vi "Set Hardware FP Connections.vi"(7 "command (Connect)":T8, 8 "error in (no error)":errorcluster, 11 "Engine Run Time Data in":T1) -> (0 "error out":errorcluster, 3 "Engine Run Time Data out":T1)   [LabVIEW 2023, in "NI 272x Resistive Simulation Custom Device Engine.lvlib"]
uses:
  NI 272x Resistive Simulation Custom Device Engine.lvlib
  <instrlib>/ni272xReferenceVIs/ni272xReferenceVIs.llb/ni272x Connector Identifier.ctl
  <instrlib>/ni272xReferenceVIs/ni272xReferenceVIs.llb/ni272x Disconnect from Connector 1Chan.vi
  <instrlib>/ni272xReferenceVIs/ni272xReferenceVIs.llb/ni272x Connect to Connector 1Chan.vi
  <instrlib>/ni272xReferenceVIs/ni272xReferenceVIs.llb/ni272x Reference.ctl
  Controls/Connection control.ctl
  Controls/Channel Mode.ctl
  NI 272x Resistive Simulation Custom Device Shared.lvlib
  <instrlib>/ni272xReferenceVIs/ni272xReferenceVIs.llb/ni272x Callendar-Van Dusen RTD Parameters.ctl
  Controls/Compiled HW Channel.ctl
  Controls/Compiled Connect Channel.ctl
  Controls/Compiled Engine Data.ctl
  Controls/Engine Run Time Data.ctl
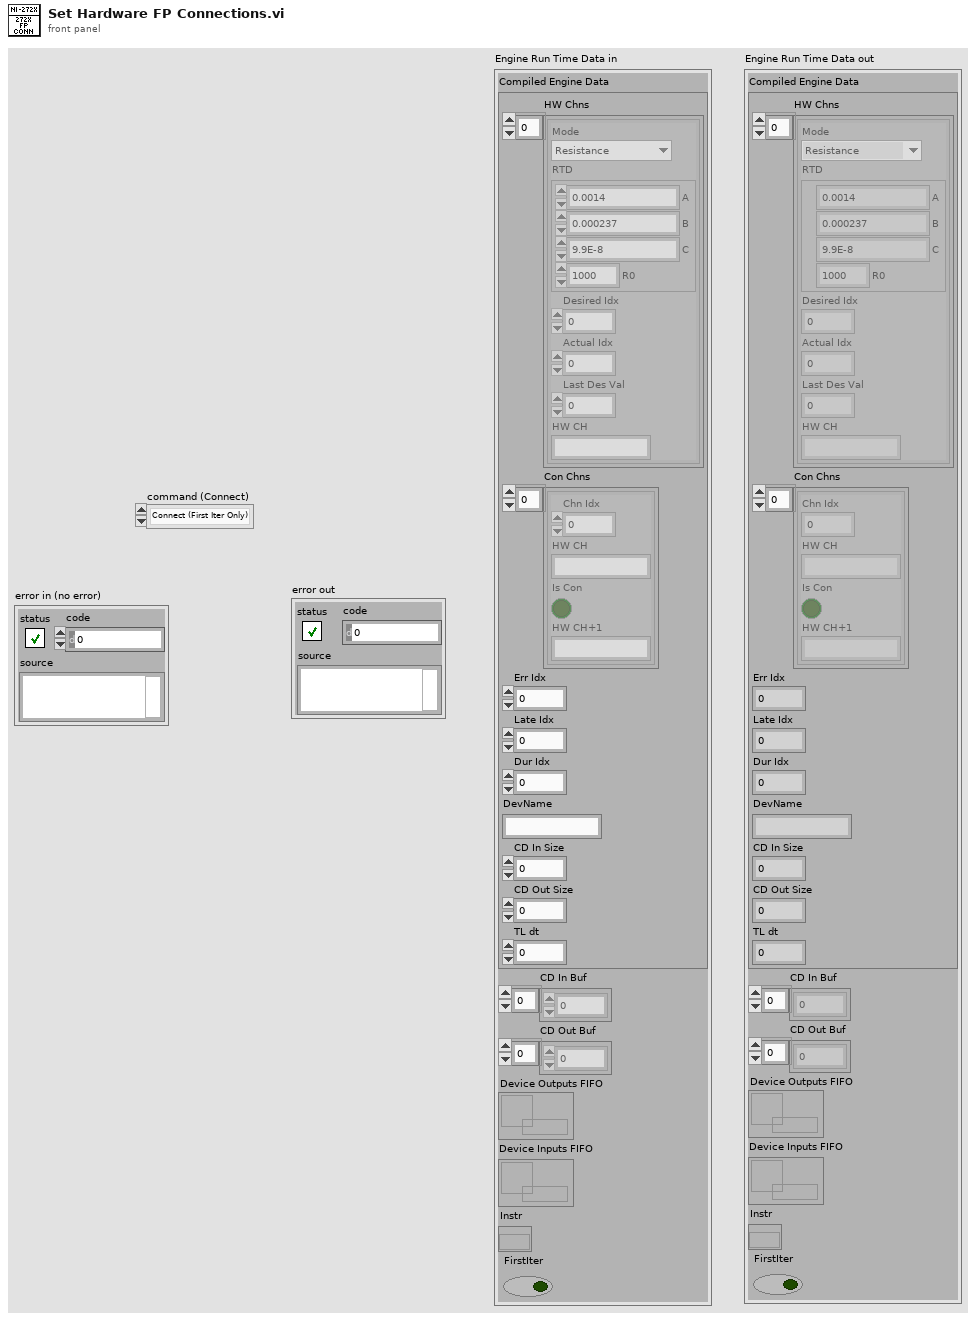
[diagram p1: front panel]
types:
  T1 = typedef "NI 272x Resistive Simulation Custom Device Engine.lvlib/Engine Run Time Data.ctl" = cluster{"Compiled Engine Data":T2, "CD In Buf":dbl[], "CD Out Buf":dbl[], "Device Outputs FIFO":refnum<k33>, "Device Inputs FIFO":refnum<k33>, "Instr":T7, "FirstIter":bool}
  T2 = typedef "NI 272x Resistive Simulation Custom Device Shared.lvlib/Compiled Engine Data.ctl" = cluster{"HW Chns":T3[], "Con Chns":T6[], "Err Idx":i32, "Late Idx":i32, "Dur Idx":i32, "DevName":string, "CD In Size":i32, "CD Out Size":i32, "TL dt":i64}
  T3 = typedef "NI 272x Resistive Simulation Custom Device Shared.lvlib/Compiled HW Channel.ctl" = cluster{"Mode":T4, "RTD":T5, "Desired Idx":i32, "Actual Idx":i32, "Last Des Val":dbl, "HW CH":string}
  T4 = typedef "NI 272x Resistive Simulation Custom Device Shared.lvlib/Channel Mode.ctl" = enum16{"Resistance", "RTD Temperature"}
  T5 = typedef "ni272x Callendar-Van Dusen RTD Parameters.ctl" = cluster{"A":dbl, "B":dbl, "C":dbl, "R0":dbl}
  T6 = typedef "NI 272x Resistive Simulation Custom Device Shared.lvlib/Compiled Connect Channel.ctl" = cluster{"Chn Idx":i32, "HW CH":string, "Is Con":bool, "HW CH+1":string}
  T7 = typedef "ni272x Reference.ctl" = refnum<k20>
  T8 = typedef "NI 272x Resistive Simulation Custom Device Engine.lvlib/Connection control.ctl" = enum16{"Connect (First Iter Only)", "Disconnect"}
  T9 = typedef "ni272x Connector Identifier.ctl" = enum8{"DUT Connector", "DMM Test Connector"}
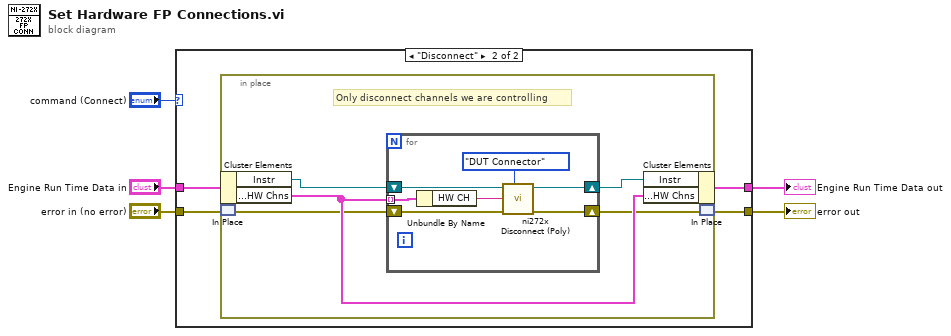
[diagram p0: block diagram]
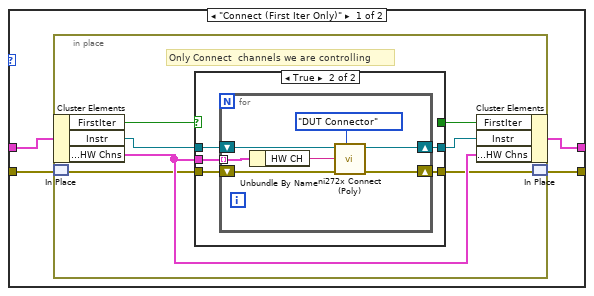
[diagram p2: hidden frame]
diagram:
  n1 = case shown="\"Disconnect\"" "command (Connect)" {
    tunnel: "error in (no error)" -> [w7 w33]
    tunnel: [w6 w32] -> w4
    tunnel: "Engine Run Time Data in" -> [w9 w35]
    tunnel: [w8 w34] -> w1
    frame "Connect (First Iter Only)" {
      n2 = in-place {
        # "Only Connect  channels we are controlling"
        n3 = in-place-cluster #1(w9) -> ("FirstIter"=w13:bool, "Instr"=w16:T7, "Compiled Engine Data.HW Chns"=w14:T3[])
        n4 = in-place-match #2(w7) -> (w11:errorcluster)
        n5 = case shown="True" w13 {
          selector: w13 -> [w17 _]
          tunnel: w11 -> [w18 w24]
          tunnel: [w18 w23] -> w10
          tunnel: w16 -> [w19 w22]
          tunnel: [w19 w21] -> w15
          tunnel: w14 -> [_ w20]
          tunnel: [w17 _] -> w12
          frame False {
          }
          frame True {
            n6 = for {
              shift-right: [w31] -> w23
              shift-left: w24 -> [w30]
              shift-right: [w28] -> w21
              shift-left: w22 -> [w29]
              tunnel: w20 -> [w26] mode=indexing
              n7 = Unbundle By Name(w26) -> ("HW CH"=w25:string)
              n8 = call-poly <instrlib>:"ni272x Connect (Poly).vi"("connector identifier"=ni272x_Connector_Identifier."DUT Connector", "error in (no error)"=w30, "resistor channel"=w25, "instrument handle"=w29) -> ("error out"=w31:errorcluster, "instrument handle out"=w28:T7)  [unwired: 6 in]
            }
          }
        }
        n9 = in-place-cluster #1("FirstIter"=w12, "Instr"=w15, "Compiled Engine Data.HW Chns"=w14) -> (w8:T1)
        n10 = in-place-match #2(w10) -> (w6:errorcluster)
      }
    }
    frame "Disconnect" {
      n11 = in-place {
        # "Only disconnect channels we are controlling"
        n12 = in-place-cluster #3(w35) -> ("Instr"=w40:T7, "Compiled Engine Data.HW Chns"=w38:T3[])
        n13 = in-place-match #4(w33) -> (w37:errorcluster)
        n14 = for {
          shift-right: [w47] -> w36
          shift-left: w37 -> [w46]
          shift-right: [w44] -> w39
          shift-left: w40 -> [w45]
          tunnel: w38 -> [w42] mode=indexing
          n15 = Unbundle By Name(w42) -> ("HW CH"=w41:string)
          n16 = call-poly <instrlib>:"ni272x Disconnect (Poly).vi"("connector identifier"=ni272x_Connector_Identifier."DUT Connector", "error in (no error)"=w46, "resistor channel"=w41, "instrument handle"=w45) -> ("error out"=w47:errorcluster, "instrument handle out"=w44:T7)  [unwired: 6 out]
        }
        n17 = in-place-cluster #3("Instr"=w39, "Compiled Engine Data.HW Chns"=w38) -> (w34:T1)
        n18 = in-place-match #4(w36) -> (w32:errorcluster)
      }
    }
  }
  "error out" <- w4
  "Engine Run Time Data out" <- w1
